vi "Team Name.vi"(11 "Team in":refnum<class "Team.lvclass">) -> (2 "Team Name":string)   [LabVIEW 2020, in "SquareBattle.lvlib" / "Team.lvclass"]
doc: "Provides the name of the team to be displayed."
uses:
  Team.lvclass
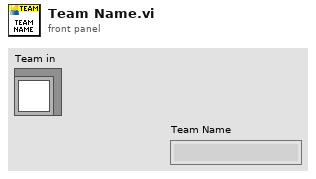
[diagram p1: front panel]
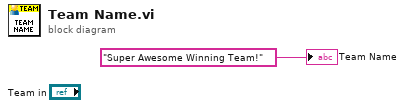
[diagram p0: block diagram]
diagram:
  "Team Name" <- "Super Awesome Winning Team!" ("Team Name")
